vi "AgPSA _Query Frequency Lock.vi"(8 "error in (no error)":errorcluster, 11 "VISA resource":refnum<visa-resource-name>) -> (0 "error out":errorcluster, 2 "Locked":bool, 3 "VISA resource":refnum<visa-resource-name>)   [LabVIEW 2015]
uses:
  <instrlib>/Agilent ESA PSA Series/Agilent ESA PSA Series.lvlib
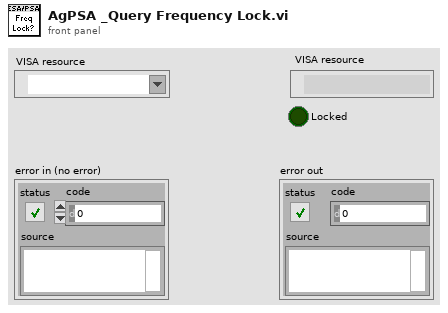
[diagram p1: front panel]
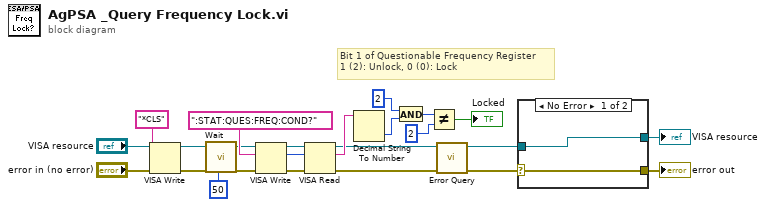
[diagram p0: block diagram]
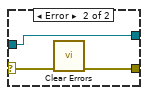
[diagram p2: hidden frame]
diagram:
  # "Bit 1 of Questionable Frequency Register\n1 (2): Unlock, 0 (0): Lock"
  n1 = VISA Write(VISA resource name="VISA resource", write buffer="*CLS", error in (no error)="error in (no error)") -> (VISA resource name out=w3:refnum<visa-resource-name>, error out=w5:errorcluster)  [unwired: 1 out]
  n2 = call "Wait.vi"("Error In"=w5, "Wait (ms)"=u32 50) -> ("Error Out"=w8:errorcluster)  [unwired: 17 in]
  n3 = VISA Write(VISA resource name=w3, write buffer=":STAT:QUES:FREQ:COND?", error in (no error)=w8) -> (VISA resource name out=w21:refnum<visa-resource-name>, return count=w23:u32, error out=w20:errorcluster)
  n4 = VISA Read(VISA resource name=w21, byte count=w23, error in (no error)=w20) -> (VISA resource name out=w16:refnum<visa-resource-name>, read buffer=w19:string, error out=w14:errorcluster)  [unwired: 1 out]
  n5 = Decimal String To Number(string=w19) -> (number=w10:i32)  [unwired: 2 in, 1 out]
  n6 = And(x=2, y=w10) -> (x .and. y?=w1:i32)
  n7 = Not Equal?(x=w1, y=2) -> (x != y?=→"Locked":bool)
  n8 = call <instrlib>:"Error Query.vi"("error in (no error)"=w14, "VISA resource name"=w16) -> ("error out"=w9:errorcluster, "VISA resource name out"=w15:refnum<visa-resource-name>)  [unwired: 6 in, 2 out]
  n9 = case shown="No Error" w9 {
    selector: w9 -> [w25 w27]
    tunnel: [w24 w26] -> w17
    tunnel: w15 -> [w24 w26]
    tunnel: [w25 w28] -> w13
    frame No Error {
    }
    frame Error {
      n10 = call <vilib>:"Clear Errors.vi"("error in (no error)"=w27) -> ("error out"=w28:errorcluster)  [unwired: 5 in, 1 out]
    }
  }
  "VISA resource" <- w17
  "error out" <- w13
